vi "Register API.vi"(8 "error in (no error)":errorcluster, 10 "API":refnum<class "API.lvclass">, 11 "APIRegistrationHandler in":refnum<class "APIRegistrationHandler.lvclass">) -> (0 "error out":errorcluster, 3 "APIRegistrationHandler out":refnum<class "APIRegistrationHandler.lvclass">)   [LabVIEW 2020, in "Volatus.lvlib" / "APIRegistrationHandler.lvclass"]
uses:
  APIRegistrationHandler.lvclass
  API/API.lvclass
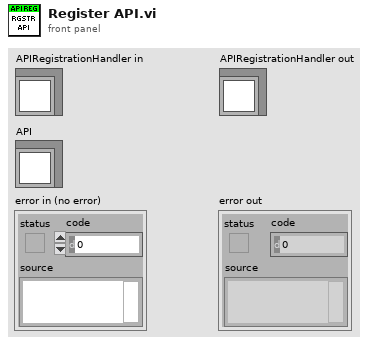
[diagram p1: front panel]
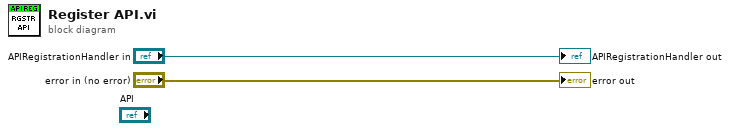
[diagram p0: block diagram]
diagram:
  "error out" <- "error in (no error)"
  "APIRegistrationHandler out" <- "APIRegistrationHandler in"
